vi "Measurement Picker.vi"(0 "discovery address":string="localhost:42000", 11 "error in":errorcluster) -> (4 "Cancelled?":bool, 6 "Measurement location":string, 8 "Measurement port":string, 13 "Measurement Name":string, 14 "Measurement Service":string, 15 "error out":errorcluster)   [LabVIEW 2020, in "InstrumentStudioPlugin_RenameMe.lvlib"]
uses:
  InstrumentStudioPlugin_RenameMe.lvlib
  <vilib>/TAF/Discovery Client/RPC Messages/NIMeasurementServices_EnumerateServicesRequest.ctl
  <vilib>/TAF/Discovery Client/RPC Messages/NIMeasurementServices_ResolveServiceRequest.ctl
  <vilib>/TAF/Discovery Client/Discovery_client.lvlib
panel:
  in  "Measurement List":i32(listbox)
  in  "Cancel":bool
  in  "OK":bool
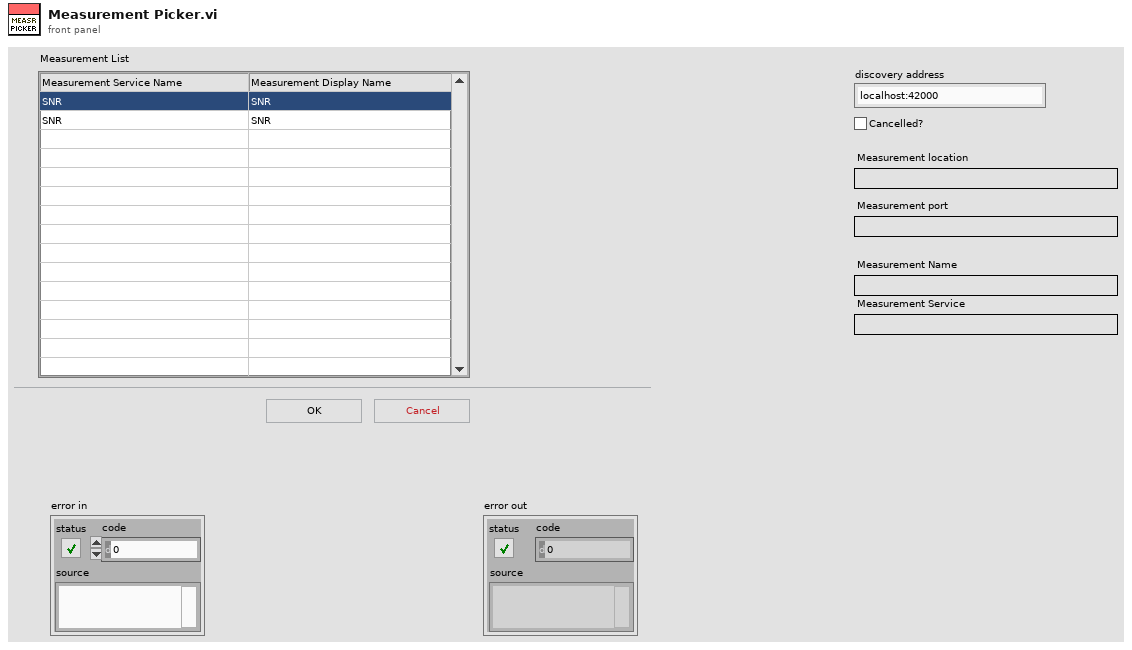
[diagram p1: front panel]
types:
  T1 = enum8{"Enabled", "Disabled", "Disabled and Grayed Out"}
  T2 = typedef "Discovery_client.lvlib/NIMeasurementServices_EnumerateServicesRequest.ctl" = cluster{"required_service":string}
  T3 = typedef "gprc-lvsupport-release.lvlib/grpcId.ctl" = u64
  T4 = typedef "Discovery_client.lvlib/NIMeasurementServices_EnumerateServicesResponse.ctl" = cluster{"available_services":T5[]}
  T5 = typedef "Discovery_client.lvlib/NIMeasurementServices_ServiceDescriptor.ctl" = cluster{"service_id":string, "name":string, "description_url":string, "service_class":string}
  T6 = typedef "Discovery_client.lvlib/NIMeasurementServices_ResolveServiceRequest.ctl" = cluster{"request_data_location":string, "required_service_class":string}
  T7 = typedef "Discovery_client.lvlib/NIMeasurementServices_ServiceLocation.ctl" = cluster{"location":string, "optimal_route":string, "insecure_port":string, "ssl_authenticated_port":string}
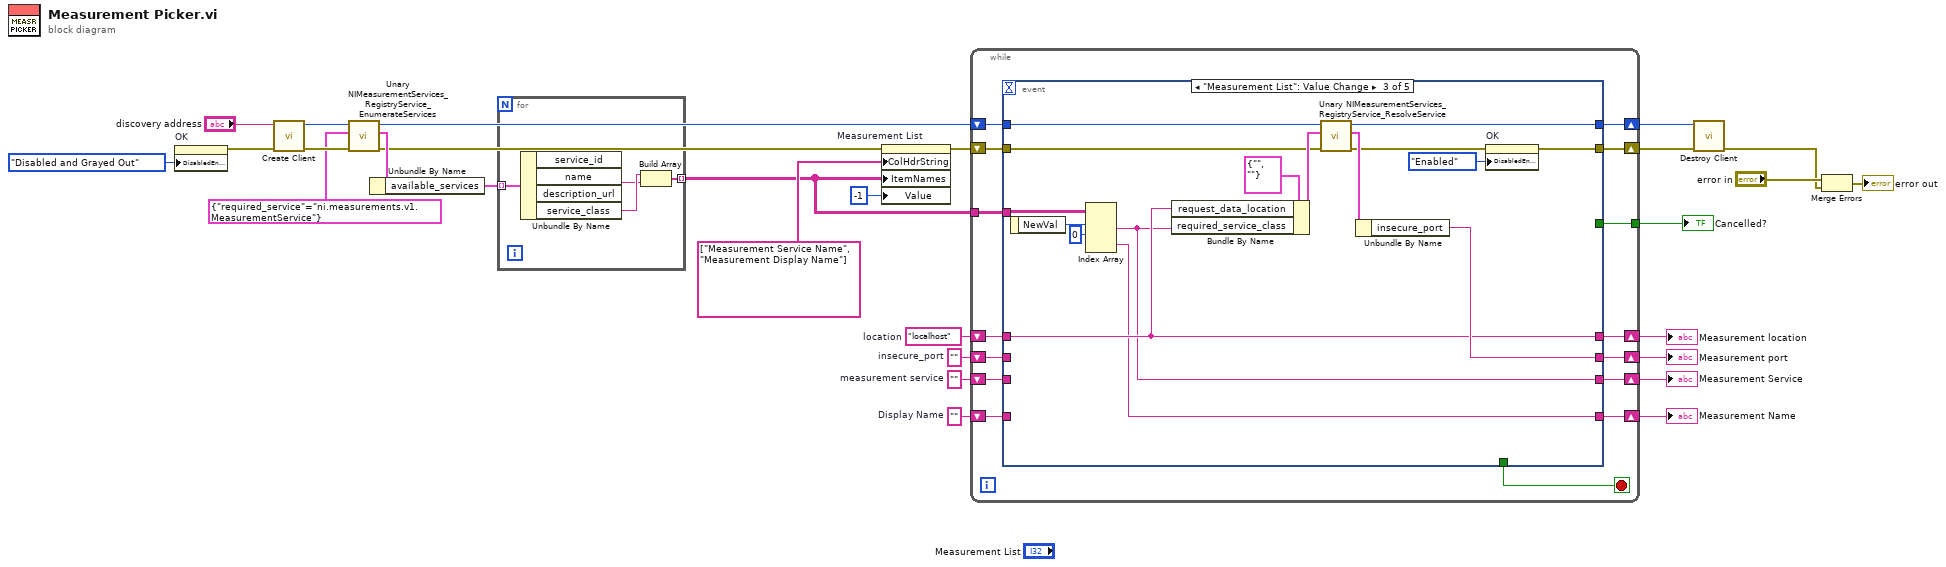
[diagram p0: block diagram]
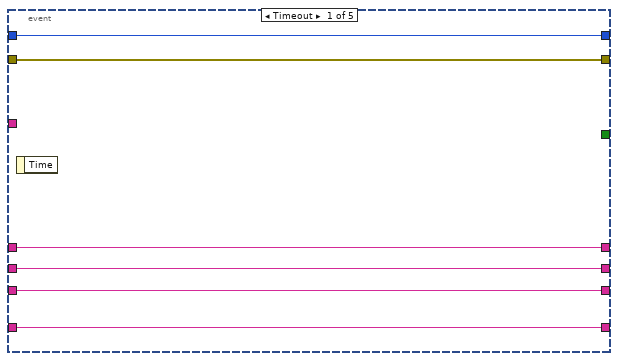
[diagram p2: hidden frame]
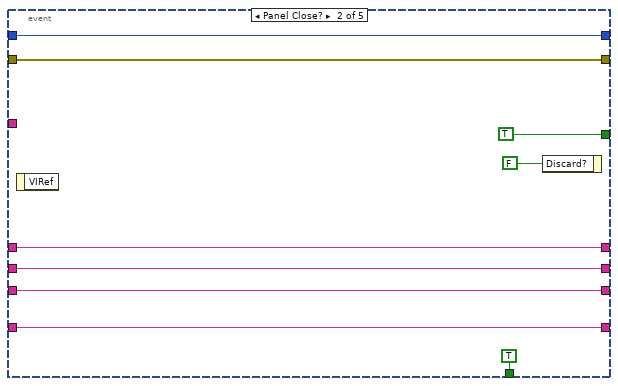
[diagram p3: hidden frame]
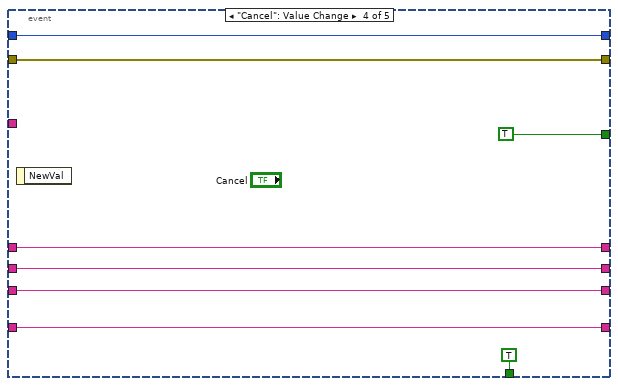
[diagram p4: hidden frame]
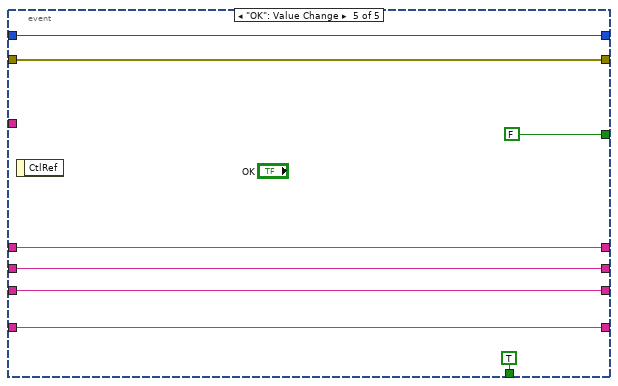
[diagram p5: hidden frame]
diagram:
  w8 = ""  # Display Name
  w9 = ""  # measurement service
  w10 = ""  # insecure_port
  w11 = "localhost"  # location
  n1 = property on="OK" class="Bool"("DisabledEnum"=T1."Disabled and Grayed Out" ("Disabled")) -> (error out=w1:errorcluster)  [unwired: 2 in, 1 out]
  n2 = call <vilib>:"Create Client.vi"("error in"=w1, "address"="discovery address") -> ("error out"=w17:errorcluster, "gRPC ID Out"=w19:T3)  [unwired: 8 in]
  n3 = call <vilib>:"Unary NIMeasurementServices_RegistryService_EnumerateServices.vi"("error in"=w17, "Request Data"=T2 {"required_service"="ni.measurements.v1.MeasurementService"}, "gRPC ID"=w19) -> ("error out"=w14:errorcluster, "Response Data"=w16:T4, "gRPC ID out"=w18:T3)  [unwired: 6 in]
  n4 = Unbundle By Name(w16) -> ("available_services"=w15:T5[])
  n5 = for {
    tunnel: w15 -> [w32] mode=indexing
    tunnel: [w29] -> w3 mode=indexing
    n6 = Unbundle By Name(w32) -> ("name"=w30:string, "service_class"=w31:string)  [unwired: 2 out]
    n7 = Build Array(w31, w30) -> (w29:string[])
  }
  n8 = property on="Measurement List" class="MCListbox (strict)"(error in=w14, "ColHdrString"=string[] ["Measurement Service Name", "Measurement Display Name"] ("Column Header Strings[]"), "ItemNames"=w3, "Value"=-1 ("Available Measurement Service")) -> (error out=w12:errorcluster)  [unwired: 1 in, 1 out]
  n9 = while {
    tunnel: [w46] -> w27
    shift-right: [w42] -> w22
    shift-left: w18 -> [w43]
    shift-right: [w41] -> w23
    shift-left: w12 -> [w40]
    tunnel: w3 -> [w39]
    shift-right: [w38] -> w6
    shift-left: w9 -> [w37]
    shift-right: [w45] -> w26
    shift-left: w11 -> [w36]
    shift-right: [w44] -> w25
    shift-left: w10 -> [w35]
    shift-right: [w34] -> w5
    shift-left: w8 -> [w33]
    stop <- w47 stop-if-true
    n10 = event shown="[2] \"Measurement List\": Value Change" {
      selector: _ -> [_ _ _ _ _]
      dyn-events: _ -> [_ _ _ _ _]
      timeout: _ -> [_ _ _ _ _]
      tunnel: [_ TRUE _ TRUE TRUE] -> w47
      tunnel: [_ TRUE _ TRUE FALSE] -> w46
      tunnel: [w50 w56 w69 w81 w89] -> w45
      tunnel: [w49 w55 w70 w80 w88] -> w44
      tunnel: w43 -> [w53 w59 w73 w84 w92]
      tunnel: [w53 w59 w72 w84 w92] -> w42
      tunnel: [w52 w58 w64 w83 w91] -> w41
      tunnel: w40 -> [w52 w58 w71 w83 w91]
      tunnel: w39 -> [_ _ w77 _ _]
      tunnel: [w51 w57 w67 w82 w90] -> w38
      tunnel: w37 -> [w51 w57 _ w82 w90]
      tunnel: w36 -> [w50 w56 w69 w81 w89]
      tunnel: w35 -> [w49 w55 _ w80 w88]
      tunnel: [w48 w54 w66 w79 w87] -> w34
      tunnel: w33 -> [w48 w54 _ w79 w87]
      event Timeout {
        n11 = event-data() -> ()  [unwired: 1 in, 1 out]
      }
      event Panel Close? {
        n12 = event-data() -> ()  [unwired: 1 in, 1 out]
        n13 = event-data("Discard?"=FALSE) -> ()  [unwired: 1 in, 1 out]
      }
      event "Measurement List": Value Change {
        n14 = event-data() -> ("NewVal"=w78:i32)  [unwired: 1 in]
        n15 = Index Array(array=w77, index (row) #1=w78, index (col) #1=0 ("disabled index (col)")) -> (element #1=w67:string, element #2=w66:string)  [unwired: 2 in]
        n16 = Bundle By Name(cluster=T6 {"request_data_location"="", "required_service_class"=""} ("Request Data"), "request_data_location"=w69, "required_service_class"=w67) -> (w76:T6)
        n17 = call <vilib>:"Unary NIMeasurementServices_RegistryService_ResolveService.vi"("error in"=w71, "Request Data"=w76, "gRPC ID"=w73) -> ("error out"=w65:errorcluster, "Response Data"=w75:T7, "gRPC ID out"=w72:T3)  [unwired: 6 in]
        n18 = Unbundle By Name(w75) -> ("insecure_port"=w70:string)
        n19 = property on="OK" class="Bool"(error in=w65, "DisabledEnum"=T1."Enabled" ("Disabled")) -> (error out=w64:errorcluster)  [unwired: 1 in, 1 out]
      }
      event "Cancel": Value Change {
        n20 = event-data() -> ()  [unwired: 1 in, 1 out]
      }
      event "OK": Value Change {
        n21 = event-data() -> ()  [unwired: 1 in, 1 out]
      }
    }
  }
  "Cancelled?" <- w27
  "Measurement location" <- w26
  "Measurement port" <- w25
  "Measurement Name" <- w5
  "Measurement Service" <- w6
  n22 = call <vilib>:"Destroy Client.vi"("error in"=w23, "gRPC ID"=w22) -> ("error out"=w20:errorcluster)  [unwired: 9 in]
  n23 = Merge Errors("error in", w20) -> (→"error out":errorcluster)
